vi "EIP Write Tags.vi"(4 "Previous Values buffer":cluster{"Tag Values":dbl[]}[](array[cluster]), 6 "Tag Data":T4[](array[typedef]) {"Device Reference" format="%.0x"}, 7 "Device Settings":T2, 8 "error in":errorcluster, 9 "Session In":T1, 10 "Device Inputs In":dbl[](array[numeric]), 11 "Device Inputs FIFO":refnum<k33>) -> (0 "error out":errorcluster, 1 "Session Out":T1, 2 "Device Inputs Out":dbl[](array[numeric]))   [LabVIEW 2023, in "Ethernet IP Custom Device Custom Device.lvlib"]
uses:
  Ethernet IP Custom Device Custom Device.lvlib
  EIP Tag Information.ctl
  <vilib>/NI VeriStand/Custom Device API/Custom Device Item Info.ctl
  <vilib>/NI VeriStand/Custom Device API/Custom Device Item Ref.ctl
  L5K Data Types.ctl
  EIP Attribute Channel Info.ctl
  EIP Attribute Direction.ctl
  EIP Device Settings.ctl
  EIP Message Type.ctl
  <vilib>/ethernetip/ethernetip.llb/ethernetip.ctl
  <vilib>/ethernetip/ethernetip.llb/EthernetIP Tag Write SINT.vi
  <vilib>/ethernetip/ethernetip.llb/EthernetIP Tag Write INT.vi
  <vilib>/ethernetip/ethernetip.llb/EthernetIP Tag Write DINT.vi
  <vilib>/ethernetip/ethernetip.llb/EthernetIP Tag Write REAL.vi
  <vilib>/ethernetip/ethernetip.llb/EthernetIP Tag Write BOOL.vi
  <vilib>/ethernetip/ethernetip.lvlib
  <vilib>/NI VeriStand/Custom Device API/Custom Device API.lvlib
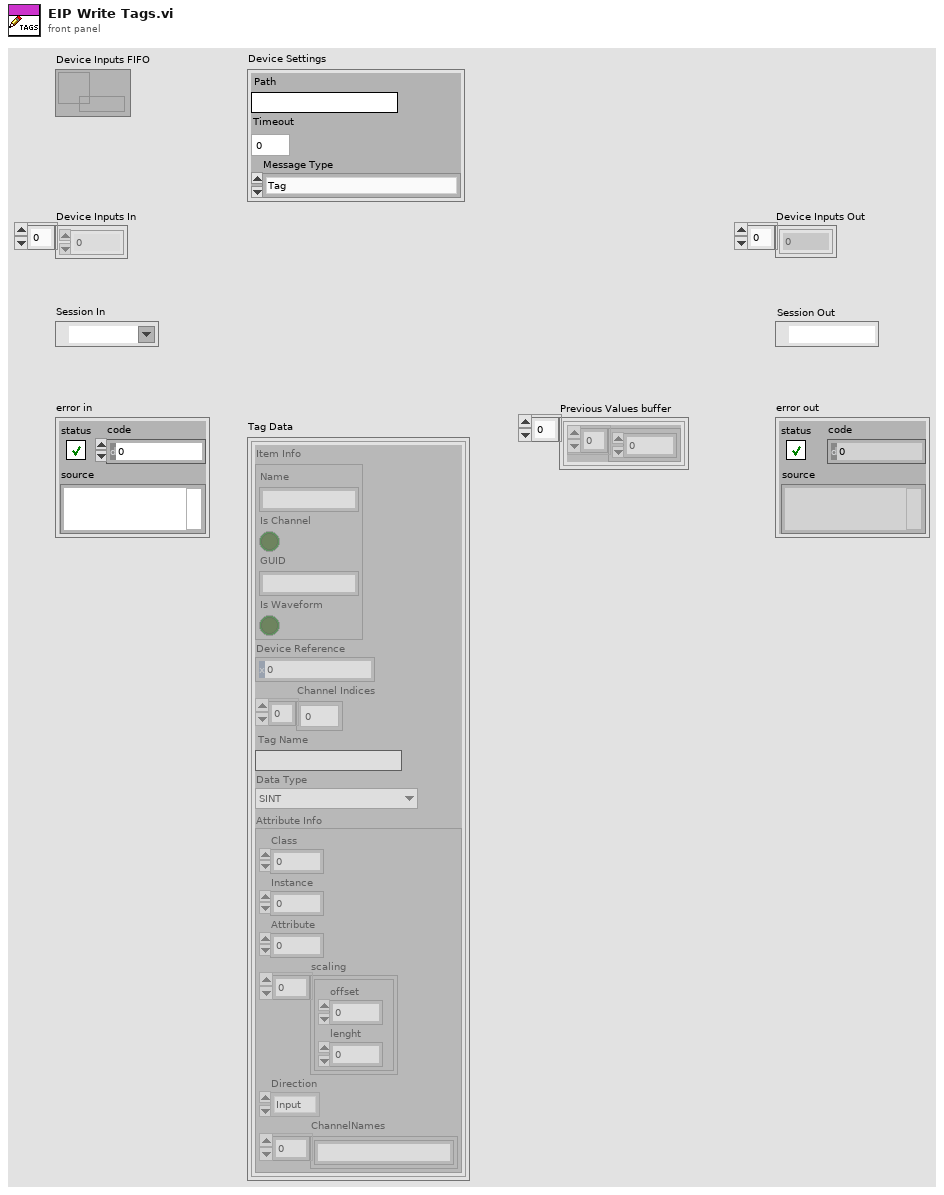
[diagram p1: front panel]
types:
  T1 = typedef "ethernetip.lvlib/ethernetip.ctl" = refnum<k21>
  T2 = typedef "Ethernet IP Custom Device Custom Device.lvlib/EIP Device Settings.ctl" = cluster{"Path":string, "Timeout":i32, "Message Type":T3}
  T3 = typedef "Ethernet IP Custom Device Custom Device.lvlib/EIP Message Type.ctl" = enum16{"Tag", "Assembly"}
  T4 = typedef "Ethernet IP Custom Device Custom Device.lvlib/EIP Tag Information.ctl" = cluster{"Item Info":T5, "Device Reference":T6, "Channel Indices":i32[], "Tag Name":string, "Data Type":T7, "Attribute Info":T8}
  T5 = typedef "Custom Device API.lvlib/Custom Device Item Info.ctl" = cluster{"Name":string, "Is Channel":bool, "GUID":string, "Is Waveform":bool}
  T6 = typedef "Custom Device API.lvlib/Custom Device Item Ref.ctl" = u64
  T7 = typedef "Ethernet IP Custom Device Custom Device.lvlib/L5K Data Types.ctl" = enum16{"SINT", "INT", "DINT", "REAL", "BOOL"}
  T8 = typedef "Ethernet IP Custom Device Custom Device.lvlib/EIP Attribute Channel Info.ctl" = cluster{"Class":i32, "Instance":u32, "Attribute":i32, "scaling":cluster{"offset":u32, "lenght":u32}[], "Direction":T9, "ChannelNames":string[]}
  T9 = typedef "Ethernet IP Custom Device Custom Device.lvlib/EIP Attribute Direction.ctl" = enum16{"Input", "Output"}
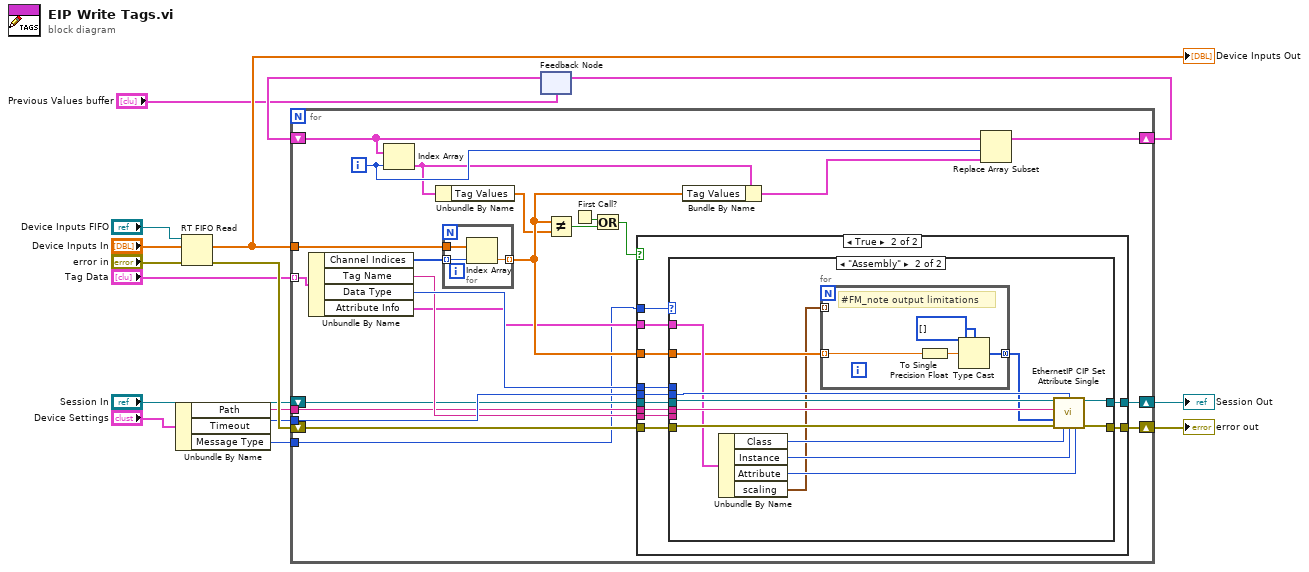
[diagram p0: block diagram]
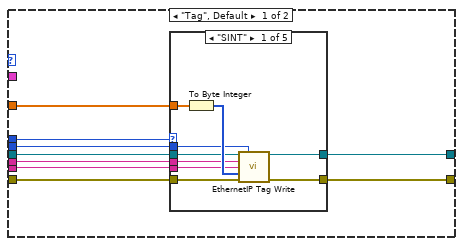
[diagram p3: hidden frame]
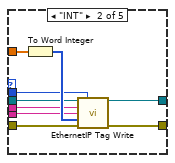
[diagram p4: hidden frame]
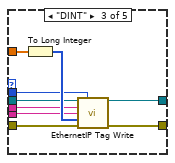
[diagram p5: hidden frame]
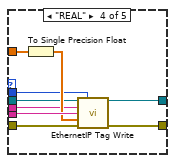
[diagram p6: hidden frame]
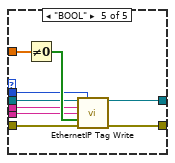
[diagram p7: hidden frame]
diagram:
  n1 = Unbundle By Name("Device Settings") -> ("Path"=w11:string, "Timeout"=w10:i32, "Message Type"=w1:T3)
  n2 = RT FIFO Read(0:"Device Inputs FIFO", 1:"Device Inputs In", 3:"error in") -> (9:w8:dbl[], 11:w13:errorcluster)  [unwired: 1 in, 3 out]
  "Device Inputs Out" <- w8
  n3 = feedback #1("Previous Values buffer") -> (w4:cluster{"Tag Values":dbl[]}[])
  n4 = for {
    tunnel: w8 -> [w38]
    shift-right: [w34] -> w7
    shift-left: w13 -> [w35]
    tunnel: w11 -> [w31]
    tunnel: w10 -> [w33]
    tunnel: "Tag Data" -> [w39] mode=indexing
    shift-right: [w29] -> w5
    shift-left: "Session In" -> [w30]
    shift-right: [w24] -> w2
    shift-left: w4 -> [w28]
    tunnel: w1 -> [w17]
    i -> [w27]
    n5 = Unbundle By Name(w39) -> ("Channel Indices"=w37:i32[], "Tag Name"=w32:string, "Data Type"=w36:T7, "Attribute Info"=w18:T8)
    n6 = Index Array(array=w28, index=w27) -> (element=w26:cluster{"Tag Values":dbl[]})
    n7 = Unbundle By Name(w26) -> ("Tag Values"=w22:dbl[])
    n8 = for {
      tunnel: w38 -> [w124]
      tunnel: w37 -> [w126] mode=indexing
      tunnel: [w125] -> w23 mode=indexing
      n9 = Index Array(array=w124, index=w126) -> (element=w125:dbl)
    }
    n10 = Not Equal?(x=w23, y=w22) -> (x != y?=w21:bool)
    n11 = First Call?() -> (First Call?: T/F=w20:bool)
    n12 = Or(x=w20, y=w21) -> (x .or. y?=w19:bool)
    n13 = case shown="True" w19 {
      tunnel: w36 -> [_ w52]
      tunnel: w35 -> [w40 w51]
      tunnel: [w40 w50] -> w34
      tunnel: w33 -> [_ w49]
      tunnel: w32 -> [_ w48]
      tunnel: w31 -> [_ w47]
      tunnel: w30 -> [w41 w46]
      tunnel: [w41 w45] -> w29
      tunnel: w23 -> [_ w44]
      tunnel: w17 -> [_ w43]
      tunnel: w18 -> [_ w42]
      frame False {
      }
      frame True {
        n14 = case shown="\"Assembly\"" w43 {
          tunnel: w52 -> [w61 _]
          tunnel: w51 -> [w60 w114]
          tunnel: [w59 w118] -> w50
          tunnel: w49 -> [w58 w117]
          tunnel: w48 -> [w57 _]
          tunnel: w47 -> [w56 w115]
          tunnel: w46 -> [w55 w116]
          tunnel: [w54 w119] -> w45
          tunnel: w44 -> [w53 w109]
          tunnel: w42 -> [_ w113]
          frame "Tag", Default {
            n15 = case shown="\"SINT\"" w61 {
              tunnel: w57 -> [w68 w77 w86 w97 w104]
              tunnel: w53 -> [w70 w79 w88 w96 w106]
              tunnel: w56 -> [w65 w73 w83 w92 w101]
              tunnel: w58 -> [w64 w74 w82 w91 w100]
              tunnel: w60 -> [w67 w76 w85 w94 w103]
              tunnel: [w66 w75 w84 w93 w102] -> w59
              tunnel: w55 -> [w62 w71 w81 w90 w98]
              tunnel: [w63 w72 w80 w89 w99] -> w54
              frame "SINT" {
                n16 = To Byte Integer(number=w70) -> (8bit integer=w69:i8[])
                n17 = call-poly <vilib>:"EthernetIP Tag Write.vi"("Session in"=w62, "Timeout (ms)"=w64, "Network Path"=w65, "Tag Name"=w68, "Data"=w69, "error in"=w67) -> ("Session out"=w63:T1, "error out"=w66:errorcluster)  [unwired: 8 in]
              }
              frame "INT" {
                n18 = To Word Integer(number=w79) -> (16bit integer=w78:i16[])
                n19 = call-poly <vilib>:"EthernetIP Tag Write.vi"("Session in"=w71, "Timeout (ms)"=w74, "Network Path"=w73, "Tag Name"=w77, "Data"=w78, "error in"=w76) -> ("Session out"=w72:T1, "error out"=w75:errorcluster)  [unwired: 8 in]
              }
              frame "DINT" {
                n20 = To Long Integer(number=w88) -> (32bit integer=w87:i32[])
                n21 = call-poly <vilib>:"EthernetIP Tag Write.vi"("Session in"=w81, "Timeout (ms)"=w82, "Network Path"=w83, "Tag Name"=w86, "Data"=w87, "error in"=w85) -> ("Session out"=w80:T1, "error out"=w84:errorcluster)  [unwired: 8 in]
              }
              frame "REAL" {
                n22 = To Single Precision Float(number=w96) -> (single precision float=w95:sgl[])
                n23 = call-poly <vilib>:"EthernetIP Tag Write.vi"("Session in"=w90, "Timeout (ms)"=w91, "Network Path"=w92, "Tag Name"=w97, "Data"=w95, "error in"=w94) -> ("Session out"=w89:T1, "error out"=w93:errorcluster)  [unwired: 8 in]
              }
              frame "BOOL" {
                n24 = Not Equal To 0?(x=w106) -> (x != 0?=w105:bool[])
                n25 = call-poly <vilib>:"EthernetIP Tag Write.vi"("Session in"=w98, "Timeout (ms)"=w100, "Network Path"=w101, "Tag Name"=w104, "Data"=w105, "error in"=w103) -> ("Session out"=w99:T1, "error out"=w102:errorcluster)  [unwired: 8 in]
              }
            }
          }
          frame "Assembly" {
            n26 = Unbundle By Name(w113) -> ("Class"=w112:i32, "Instance"=w111:u32, "Attribute"=w110:i32, "scaling"=w108:cluster{"offset":u32, "lenght":u32}[])
            n27 = for {
              tunnel: w109 -> [w122] mode=indexing
              tunnel: w108 -> [_] mode=indexing
              tunnel: [w120] -> w107 mode=concatenating
              # "#FM_note output limitations"
              n28 = To Single Precision Float(number=w122) -> (single precision float=w121:sgl)
              n29 = Type Cast(type=u8[] [] ("Data"), x=w121) -> (*(type *) &x=w120:u8[])
            }
            n30 = call <vilib>:"EthernetIP CIP Set Attribute Single.vi"("Session in"=w116, "Timeout (ms)"=w117, "Network Path"=w115, "Data"=w107, "error in"=w114, "Class"=w112, "Instance"=w111, "Attribute"=w110) -> ("Session out"=w119:T1, "error out"=w118:errorcluster)  [unwired: 6 in]
          }
        }
      }
    }
    n31 = Bundle By Name(cluster=w26, "Tag Values"=w23) -> (w25:cluster{"Tag Values":dbl[]})
    n32 = Replace Array Subset(array=w28, new element=w25, index=w27) -> (w24:cluster{"Tag Values":dbl[]}[])
  }
  "error out" <- w7
  "Session Out" <- w5
  n33 = feedback-in #1(w2) -> ()
